vi "io.init.vi"   [LabVIEW 2019]
uses:
  <vilib>/rvi/eio/common/nirviEmuTemplateMethod_errors.vi
  <vilib>/eio/EIOMethodNode/EIOMethodNode.xnode
types:
  T1 = enum8{"NOP", "Commutation", "Acceleration", "Commut. & Acceler.", "Marginality Signal", "Marginality & Acceler.", "Asynchr. Pos Value 1 (LSB)", "Asynchr. Pos Value 2", "Asynchr. Pos Value 3 (MSB)", "Operating State Error", "Unused", "timestamp", "Reserved1", "Reserved2", "Reserved3", "Stop Sending Info2"}
  T2 = enum8{"NOP", "Diagnosis", "Abs. Position Value 1 (LSB)", "Abs. Position Value 2", "Abs. Position Value 3 (MSB)", "Ackn. Memory Param. (LSB)", "Ackn. Memory Param. (MSB)", "Acknowledge MRS code", "Ackn. Test Command", "Send Test Value 1 (LSB)", "Send Test Value 2", "Send Test Value 3 (MSB)", "Temperature Sensor1", "Temperature Sensor2", "Addtl. Sensors", "Stop Sending Info1"}
  T3 = enum8{"8 MHz", "4 MHz", "2 MHz", "1 MHz", "200 kHz", "100 kHz"}
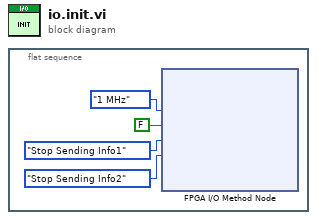
[diagram p0: block diagram]
diagram:
  n1 = flat-sequence {
    frame #0 {
      n2 = xnode "FPGA I/O Method Node"("Bus Speed"=T3."1 MHz", "Enable Add Info"=FALSE, "Add Info1"=T2."Stop Sending Info1", "Add Info2"=T1."Stop Sending Info2") -> ()  [unwired: 1 in, 3 out]
    }
  }
